vi "DB Tools Close Connection.vi"(4 "error in (no error)":errorcluster, 7 "connection reference":T1) -> (0 "error out":errorcluster)   [LabVIEW 2012, in "NI_Database_API_64.lvlib"]
doc: "Closes a database connection by destroying its associated <B>connection reference</B>."
uses:
  NI_Database_API_64.lvlib
  Conn ObjectReference.ctl
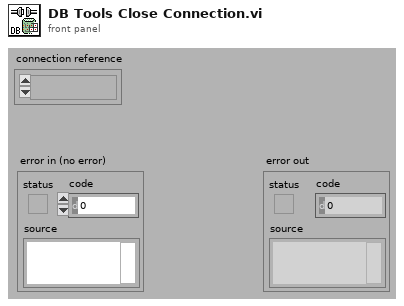
[diagram p1: front panel]
types:
  T1 = typedef "NI_Database_API_64.lvlib/Conn ObjectReference.ctl" = refnum<k1>
  T2 = typedef "NI_Database_API_64.lvlib/Conn DataMembers.ctl" = cluster{"ADODB._Connection":refnum<k7>, "recordset objects":i32, "command objects":i32}
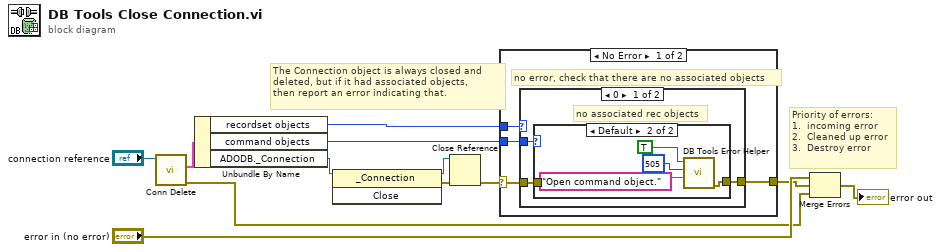
[diagram p0: block diagram]
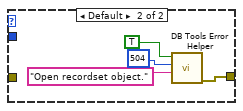
[diagram p3: hidden frame]
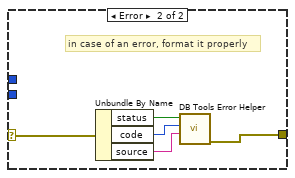
[diagram p4: hidden frame]
diagram:
  # "Priority of errors:\n1.  incoming error\n2.  Cleaned up error\n3.  Destroy error"
  # "The Connection object is always closed and \ndeleted, but if it had associated objects, \nthen report an error indicating that."
  n1 = call "Conn Delete.vi"("connection reference"="connection reference") -> ("error out"=w1:errorcluster, "data"=w12:T2)  [unwired: 1 in, 4 out]
  n2 = Unbundle By Name(w12) -> ("recordset objects"=w10:i32, "command objects"=w9:i32, "ADODB._Connection"=w8:refnum<k7>)
  n3 = invoke class="_Connection" method="Close"(reference=w8) -> (reference out=w6:refnum<k7>, error out=w7:errorcluster)  [unwired: 2 in, 1 out]
  n4 = Close Reference(reference=w6, error in (no error)=w7) -> (error out=w3:errorcluster)
  n5 = case shown="No Error" w3 {
    selector: w3 -> [w14 w30]
    tunnel: w10 -> [w16 _]
    tunnel: w9 -> [w13 _]
    tunnel: [w15 w31] -> w2
    frame No Error {
      # "no error, check that there are no associated objects"
      n6 = case shown="0" w16 {
        tunnel: [w19 w27] -> w15
        tunnel: w14 -> [w18 _]
        tunnel: w13 -> [w17 _]
        frame 0 {
          # "no associated rec objects"
          n7 = case shown="Default" w17 {
            tunnel: [w20 w23] -> w19
            tunnel: w18 -> [w20 _]
            frame 0 {
              # "no associated com objects"
            }
            frame Default {
              n8 = call "DB Tools Error Helper.vi"("source"="Open command object.", "code"=505, "status"=TRUE) -> ("error out"=w23:errorcluster)  [unwired: 1 in, 7 out]
            }
          }
        }
        frame Default {
          n9 = call "DB Tools Error Helper.vi"("source"="Open recordset object.", "code"=504, "status"=TRUE) -> ("error out"=w27:errorcluster)  [unwired: 1 in, 7 out]
        }
      }
    }
    frame Error {
      # "in case of an error, format it properly"
      n10 = Unbundle By Name(w30) -> ("status"=w33:bool, "code"=w29:i32, "source"=w32:string)
      n11 = call "DB Tools Error Helper.vi"("source"=w32, "code"=w29, "status"=w33) -> ("error out"=w31:errorcluster)  [unwired: 1 in, 7 out]
    }
  }
  n12 = Merge Errors("error in (no error)", w2, w1) -> (→"error out":errorcluster)
